vi "SubVI_bias.vi"(10 "Vector c":fxp<+/-,32,16>[](array[numeric])=[0.0, 0.0, 0.0, 0.0, 0.0, 0.0, 0.0, 0.0, 0.0, 0.0, 0.0, 0.0, 0.0, 0.0, 0.0, 0.0, 0.0, 0.0, 0.0, 0.0, 0.0, 0.0, 0.0, 0.0, 0.0, 0.0, 0.0, 0.0, 0.0, 0.0, 0.0, 0.0, 0.0, 0.0, 0.0, 0.0, 0.0, 0.0, 0.0, 0.0], 11 "Refnum in":refnum<k21>) -> (3 "Array":fxp<+/-,32,16>[](array[numeric]))   [LabVIEW 2020]
uses:
  <vilib>/rvi/DataTransferAndStorage/Container/Common/niFpgaContainerExecOnDevCompGetState.vi
  <vilib>/rvi/Emulation/niFpgaEmulationIsFPGAContextNoSignature.vi
  <vilib>/rvi/DataTransferAndStorage/Container/Common/niFpgaContainerGetUniqueNameForEmu.vi
  <vilib>/rvi/Emulation/niFpgaProcessEmulError.vi
  <vilib>/rvi/Emulation/niFpgaSctlEmulationGetInTimedLoop.vi
  <vilib>/rvi/errors/nirviReportUnexpectedCaseInternalError (U32).vi
  <vilib>/rvi/Memory/Memory_Emulation/niFpgaMemoryEmulationCacheClearOnFirstRun.vi
  <vilib>/rvi/Memory/Memory_Emulation/nirvimemoryEmulationManagerCache_MakeExclusive.vi
  <vilib>/rvi/Memory/Memory_Emulation/niFpgaMemoryEmulationValidateCache.vi
  <vilib>/rvi/Memory/Memory_Emulation/nirvimemoryEmulationManagerCache_InsertValue.vi
  <vilib>/Utility/error.llb/Clear Errors.vi
  <vilib>/rvi/Memory/Memory_Emulation/nirvimemoryEmulationManagerCache_ReleaseExclusive.vi
  <vilib>/rvi/Memory/Memory_Emulation/nirvimemoryEmulationManagerCache_GetValue.vi
  <vilib>/rvi/Memory/Memory_Emulation/nirvimemoryEmulationManagerCache_SetValue.vi
  <vilib>/rvi/Emulation/niFpgaSctlEmulationResourceMgr.vi
  <vilib>/rvi/DataTransferAndStorage/Container/XNode/niFpgaContainer.xnode
  <vilib>/rvi/Memory/Memory_Emulation/niFpgaMemoryEmulationRefIn.vi
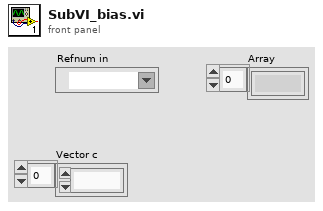
[diagram p1: front panel]
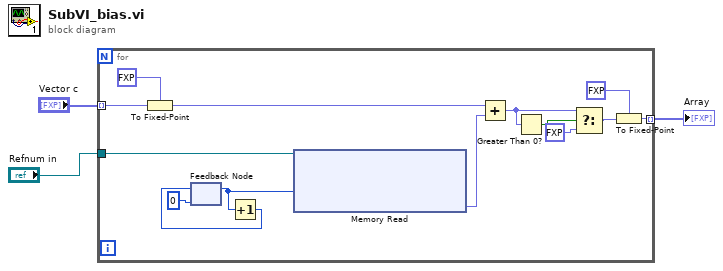
[diagram p0: block diagram]
diagram:
  n1 = for {
    tunnel: "Vector c" -> [w9] mode=indexing
    tunnel: [w5] -> w2 mode=indexing
    tunnel: "Refnum in" -> [w4]
    n2 = To Fixed-Point(fixed-point type=fxp<+/-,32,16> 0.0 ("f"), number=w9) -> (fixed-point=w13:fxp<+/-,32,16>)
    n3 = feedback #1(u32 0 ("Timeout")) -> (w12:u32)
    n4 = Increment(x=w12) -> (x+1=w11:u32)
    n5 = feedback-in #1(w11) -> ()
    n6 = xnode ("Memory Read")("Address"=w12, "Memory In"=w4) -> ("Data"=w10:fxp<+/-,32,16>)  [unwired: 1 out]
    n7 = Add(x=w13, y=w10) -> (x+y=w15:fxp<+/-,33,17>)
    n8 = Greater Than 0?(x=w15) -> (x > 0?=w17:bool)
    n9 = Select(t=w15, s=w17, f=fxp<+/-,33,17> 0.0) -> (s? t:f=w6:fxp<+/-,33,17>)
    n10 = To Fixed-Point(fixed-point type=fxp<+/-,32,16> 0.0 ("f"), number=w6) -> (fixed-point=w5:fxp<+/-,32,16>)
  }
  "Array" <- w2
